vi "Digital Name Updater.vi"(8 "error in (no error)":errorcluster, 11 "Cluster In":T1) -> (0 "error out":errorcluster, 3 "Cluster Out":T1)   [LabVIEW 2018]
uses:
  Shared Controls/Range Updater.ctl
  Val Change Checker.vi
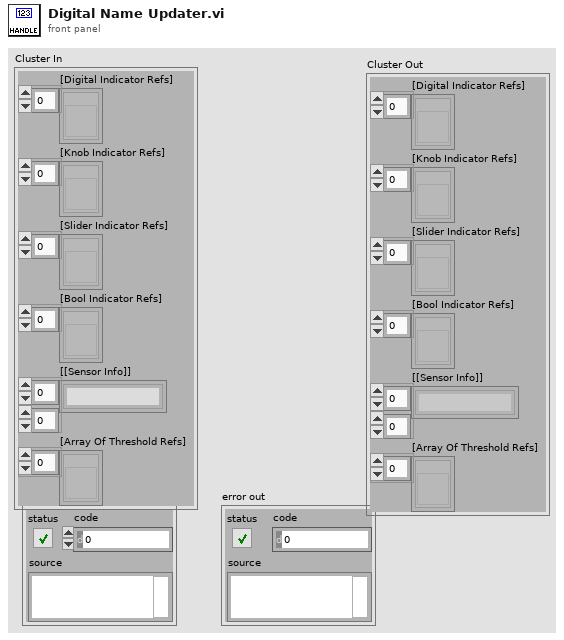
[diagram p1: front panel]
types:
  T1 = typedef "Range Updater.ctl" = cluster{"[Digital Indicator Refs]":refnum<vi>[], "[Knob Indicator Refs]":refnum<vi>[], "[Slider Indicator Refs]":refnum<vi>[], "[Bool Indicator Refs]":refnum<vi>[], "[[Sensor Info]]":string[][], "[Array Of Threshold Refs]":refnum<vi>[]}
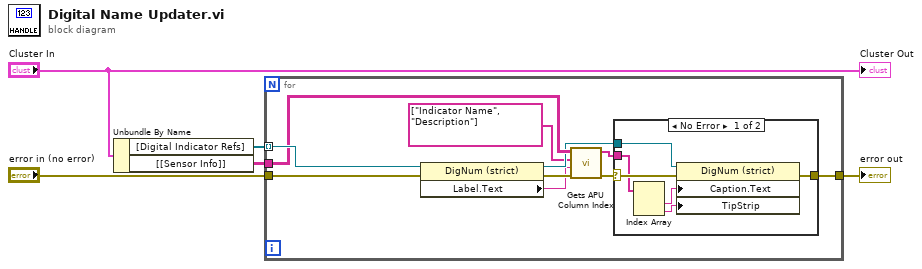
[diagram p0: block diagram]
diagram:
  n1 = Unbundle By Name("Cluster In") -> ("[Digital Indicator Refs]"=w2:refnum<vi>[], "[[Sensor Info]]"=w3:string[][])
  n2 = for {
    tunnel: w2 -> [w15] mode=indexing
    tunnel: w3 -> [w12]
    tunnel: [w13] -> w5
    tunnel: "error in (no error)" -> [w10]
    n3 = property class="DigNum (strict)"(reference=w15, error in=w10) -> (reference out=w11:refnum<vi>, error out=w14:errorcluster, "Label.Text"=w6:string)
    n4 = call "Gets APU Column Index.vi"("error in (no error)"=w14, "Tag"=w6, "[Column Names]"=string[] ["Indicator Name", "Description"], "[[Array of Info]]"=w12) -> ("error out"=w9:errorcluster, "[Values out]"=w8:string[])  [unwired: 3 in, 3 out]
    n5 = case shown="No Error" w9 {
      selector: w9 -> [w21 w22]
      tunnel: [w20 w22] -> w13
      tunnel: w11 -> [w19 _]
      tunnel: w8 -> [w18 _]
      frame No Error {
        n6 = Index Array(array=w18) -> (element #1=w17:string, element #2=w16:string)  [unwired: 2 in]
        n7 = property class="DigNum (strict)"(reference=w19, error in=w21, "Caption.Text"=w17, "TipStrip"=w16) -> (error out=w20:errorcluster)  [unwired: 1 out]
      }
      frame Error {
      }
    }
  }
  "error out" <- w5
  "Cluster Out" <- "Cluster In"
